vi "PWAtasksGLOBAL.vi"() -> ()   [LabVIEW 2013]
panel:
  out "HWReadALLinputs":refnum<k21>[](array[refnum])
  out "PWA Binary":i16[][](array[numeric])
  in  "Probe Rotated Thro' 180":bool
  in  "PWA No of Reverse samples":i32
  in  "PWA Timescales":dbl[](array[numeric]) format="%.2f"
  in  "PWA No of  TOF Below Min":i32
  in  "PWA No of  TOF Timeouts":i32
  in  "PWA Calib. File Path":path
  in  "STOP":bool
  in  "PWA Seconds per clock pulse":dbl
  in  "PWA No. of Samples":i32=100
  in  "Minimum TOF Index":i16=208
  in  "PWA Setup summary":string
  in  "PWA 1/TOF":dbl[][](array[numeric])
  in  "PWA Data":dbl[][](array[numeric])
  in  "PWA Lookup Table":dbl[](array[numeric])
  in  "PWA Symbol":string="tauw"
  in  "Software + buffering delay per pulse (s)":dbl
  in  "PWA Freq. (Hz)":dbl=20.0
  in  "PWA Dev Name":string="Dev1"
  in  "Analogue Dev Name":string="Dev2"
  out "ReadAnalogue":refnum<k21>="ReadAnalogue"
  out "ReadTOFready":refnum<k21>="ReadTOFready"
  out "BitSwitch":refnum<k21>="BitSwitch"
  out "Fire":refnum<k21>="Fire"
  out "Read1to7":refnum<k21>="Read1to7"
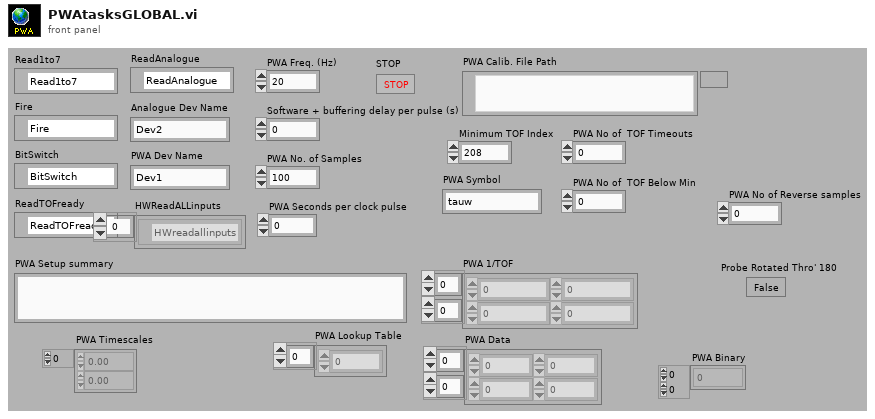
[diagram p1: front panel]
diagram:
